vi "save_list.vi"(7 "List Parameter Fit":dbl[][](array[numeric]), 9 "Elements Selected":string[][](table), 10 "list path in":path, 11 "List ROI in":dbl[][](array[numeric])) -> (2 "list path out":path, 3 "list array":string[][](array[string]))   [LabVIEW 2023]
panel:
  out "Number od ROIs":i32
  out "Number of Elements":i32
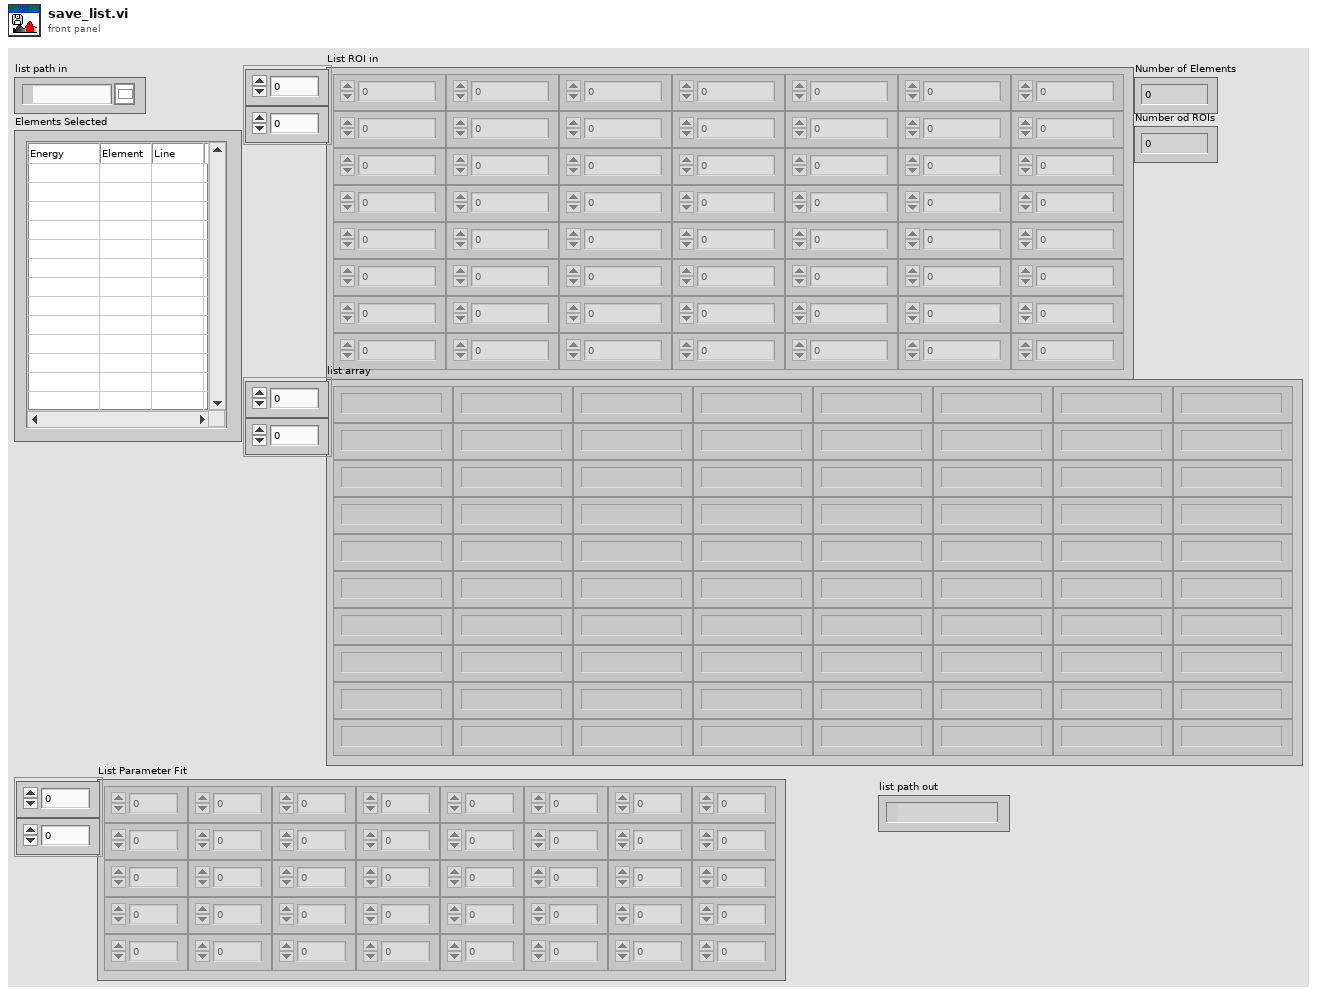
[diagram p1: front panel]
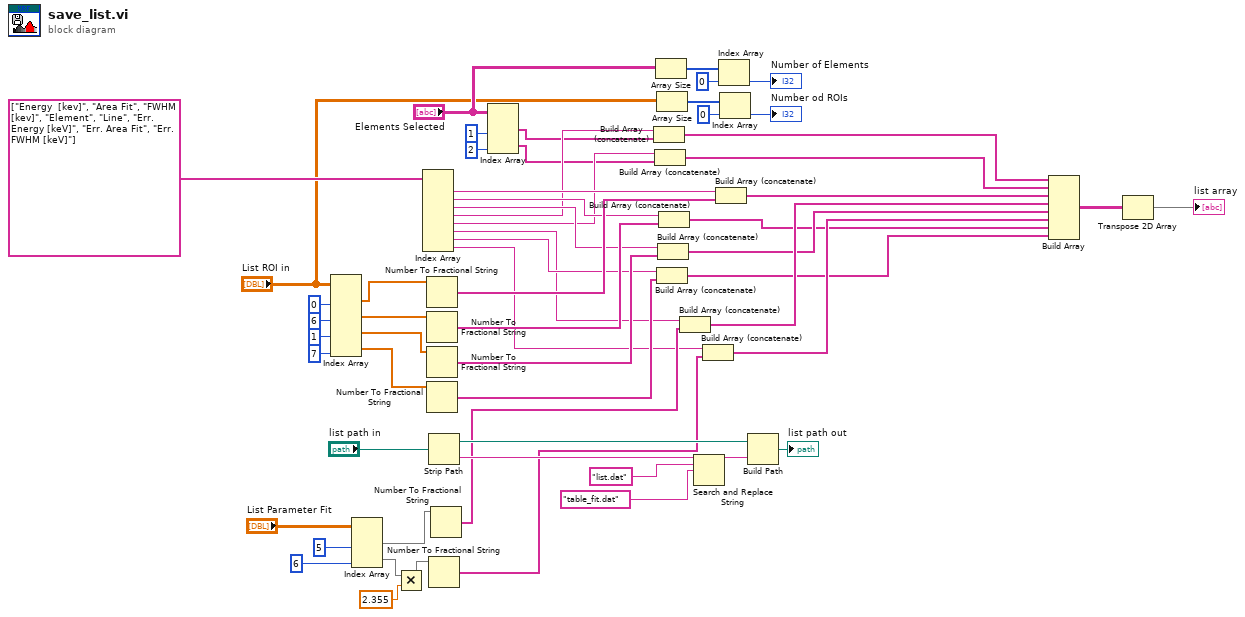
[diagram p0: block diagram]
diagram:
  n1 = Index Array(array="List ROI in", index (col) #1=0 ("disabled index (col)"), index (col) #2=6 ("index (col)"), index (col) #3=1 ("index (col)"), index (col) #4=7 ("index (col)")) -> (element #1=w56:dbl[], element #2=w55:dbl[], element #3=w54:dbl[], element #4=w22:dbl[])  [unwired: 4 in]
  n2 = Index Array(array="List Parameter Fit", index (col) #1=5 ("index (col)"), index (col) #2=6 ("index (col)")) -> (element #1=w15:dbl[], element #2=w13:dbl[])  [unwired: 2 in]
  n3 = Multiply(x=w13, y=2.355) -> (x*y=w11:dbl[])
  n4 = Index Array(array=string[] ["Energy  [kev]", "Area Fit", "FWHM [kev]", "Element", "Line", "Err. Energy [keV]", "Err. Area Fit", "Err. FWHM [keV]"]) -> (element #1=w52:string, element #2=w50:string, element #3=w48:string, element #4=w37:string, element #5=w36:string, element #6=w16:string, element #7=w20:string, element #8=w9:string)  [unwired: 8 in]
  n5 = Number To Fractional String(number=w56) -> (F-format string=w51:string[])  [unwired: 3 in]
  n6 = Number To Fractional String(number=w55) -> (F-format string=w49:string[])  [unwired: 3 in]
  n7 = Number To Fractional String(number=w54) -> (F-format string=w47:string[])  [unwired: 3 in]
  n8 = Number To Fractional String(number=w22) -> (F-format string=w21:string[])  [unwired: 3 in]
  n9 = Strip Path(path="list path in") -> (stripped path=w39:path, name=w43:string)
  n10 = Number To Fractional String(number=w11) -> (F-format string=w10:string[])  [unwired: 3 in]
  n11 = Number To Fractional String(number=w15) -> (F-format string=w14:string[])  [unwired: 3 in]
  n12 = Index Array(array="Elements Selected", index (col) #1=1 ("disabled index (col)"), index (col) #2=2 ("index (col)")) -> (element #1=w33:string[], element #2=w32:string[])  [unwired: 2 in]
  n13 = Build Array (concatenate)(w37, w33) -> (w8:string[])
  n14 = Build Array (concatenate)(w36, w32) -> (w7:string[])
  n15 = Array Size(array="Elements Selected") -> (size(s)=w30:i32[])
  n16 = Array Size(array="List ROI in") -> (size(s)=w28:i32[])
  n17 = Build Array (concatenate)(w20, w21) -> (w1:string[])
  n18 = Build Array (concatenate)(w48, w47) -> (w4:string[])
  n19 = Build Array (concatenate)(w50, w49) -> (w2:string[])
  n20 = Build Array (concatenate)(w16, w14) -> (w5:string[])
  n21 = Search and Replace String(input string=w43, search string="list.dat", replace string="table_fit.dat") -> (result string=w40:string)  [unwired: 5 in, 3 out]
  n22 = Build Array (concatenate)(w9, w10) -> (w3:string[])
  n23 = Build Array (concatenate)(w52, w51) -> (w6:string[])
  n24 = Index Array(array=w30, index=0) -> (element=→"Number of Elements":i32)
  n25 = Index Array(array=w28, index=0) -> (element=→"Number od ROIs":i32)
  n26 = Build Path(base path=w39, name or relative path=w40) -> (appended path=→"list path out":path)
  n27 = Build Array(w8, w7, w6, w5, w4, w3, w2, w1) -> (w46:string[][])
  n28 = Transpose 2D Array(2D array=w46) -> (transposed array=→"list array":string[][])
